vi "ID parser.vi"(10 "Input String":string) -> (1 "Serial":string, 2 "Model":string, 3 "Manufacturer":string)   [LabVIEW 2013, in "SetUp VIs.lvlib"]
uses:
  SetUp VIs.lvlib
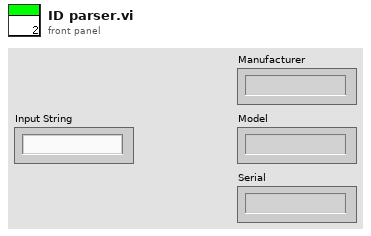
[diagram p1: front panel]
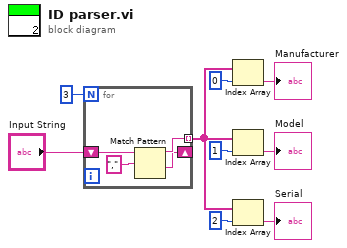
[diagram p0: block diagram]
diagram:
  n1 = for {
    N: 3 -> [_]
    tunnel: [w11] -> w2 mode=indexing
    shift-right: [w10] -> _
    shift-left: "Input String" -> [w13]
    n2 = Match Pattern(string=w13, regular expression=",") -> (before substring=w11:string, after substring=w10:string)  [unwired: 1 in, 2 out]
  }
  n3 = Index Array(array=w2, index=0) -> (element=→"Manufacturer":string)
  n4 = Index Array(array=w2, index=1) -> (element=→"Model":string)
  n5 = Index Array(array=w2, index=2) -> (element=→"Serial":string)
